vi "Tag-Get Tag.vi"(8 "error in (no error)":errorcluster, 10 "Tag Name":string, 11 "Generic in":refnum<class "Generic.lvclass">) -> (0 "error out":errorcluster, 1 "Is Persistent?":bool, 2 "Tag:Get Tag":bool, 3 "Generic out":refnum<class "Generic.lvclass">, 4 "Value":variant)   [LabVIEW 2015, in "Generic.lvclass"]
doc: "Returns a tag value associated with the tag. Returns FALSE if the tag does not exist.\n\nQControl Class wrapper around the <b>Generic : Tag:Get Tag Method</b>.\n<b> </b> <b> </b>\n©2016 Q Software Innovations, LLC (QSI)\nwritten by Quentin Alldredge\nproduced in LabVIEW 2015\n\nsupport@qsoftwareinnovations.com\nwww.qsoftwareinnovations.com\n\nAll rights reserved.\n\nRedistribution and use in source and binary forms, with or without modification, are permitted provided that the following conditions are met:\n\n * Redistributions of source code must retain the above copyright notice, this list of conditions and the following disclaimer.\n * Redistributions in binary form must reproduce the above copyright notice, this list of conditions and the following disclaimer in the documentation and/or other materials provided with the distribution.\n * Neither the name of Q Software Innovations, LLC. nor the names of its contributors may be used to endorse or promote products derived from this software without specific prior written permission.\n\nTHIS SOFTWARE IS PROVIDED BY THE COPYRIGHT HOLDERS AND CONTRIBUTORS \"AS IS\" AND ANY EXPRESS OR IMPLIED WARRANTIES, INCLUDING, BUT NOT LIMITED TO, THE IMPLIED WARRANTIES OF MERCHANTABILITY AND FITNESS FOR A PARTICULAR PURPOSE ARE DISCLAIMED. IN NO EVENT SHALL THE COPYRIGHT OWNER OR CONTRIBUTORS BE LIABLE FOR ANY DIRECT, INDIRECT, INCIDENTAL, SPECIAL, EXEMPLARY, OR CONSEQUENTIAL DAMAGES (INCLUDING, BUT NOT LIMITED TO, PROCUREMENT OF SUBSTITUTE GOODS OR SERVICES; LOSS OF USE, DATA, OR PROFITS; OR BUSINESS INTERRUPTION) HOWEVER CAUSED AND ON ANY THEORY OF LIABILITY, WHETHER IN CONTRACT, STRICT LIABILITY, OR TORT (INCLUDING NEGLIGENCE OR OTHERWISE) ARISING IN ANY WAY OUT OF THE USE OF THIS SOFTWARE, EVEN IF ADVISED OF THE POSSIBILITY OF SUCH DAMAGE."
uses:
  Generic.lvclass
  Generic.lvclass/Generic.ctl
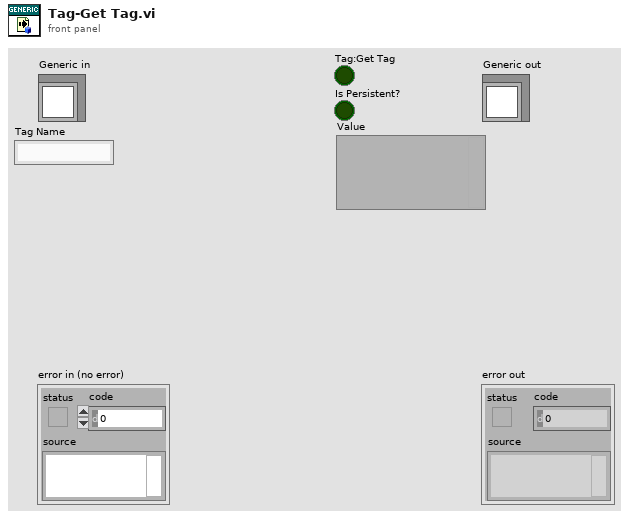
[diagram p1: front panel]
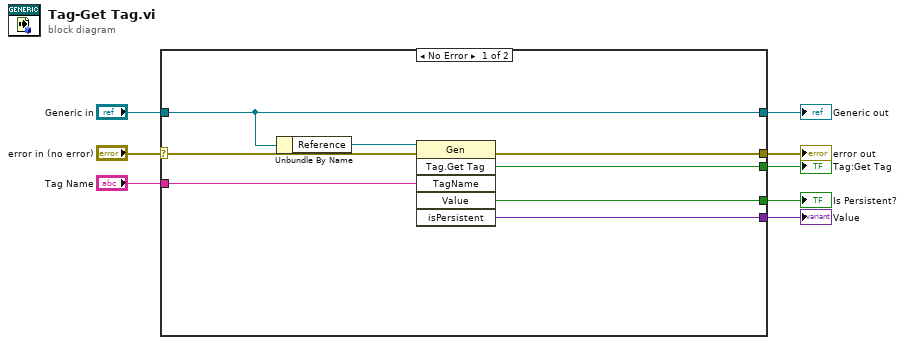
[diagram p0: block diagram]
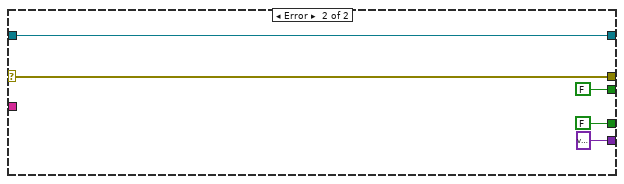
[diagram p2: hidden frame]
diagram:
  n1 = case shown="No Error" "error in (no error)" {
    selector: "error in (no error)" -> [w16 w21]
    tunnel: [w15 w21] -> w7
    tunnel: [w14 w20] -> w5
    tunnel: "Generic in" -> [w14 w20]
    tunnel: "Tag Name" -> [w12 _]
    tunnel: [w11 FALSE ("GetTag")] -> w3
    tunnel: [w10 FALSE ("Value")] -> w2
    tunnel: [w9 variant ("isPersistent")] -> w1
    frame No Error {
      n2 = Unbundle By Name(w14) -> ("Reference"=w13:refnum<vi>)
      n3 = invoke class="Gen" method="Tag.Get Tag"(reference=w13, error in=w16, "TagName"=w12) -> (error out=w15:errorcluster, "GetTag"=w11:bool, "Value"=w10:bool, "isPersistent"=w9:variant)  [unwired: 3 in, 2 out]
    }
    frame Error {
    }
  }
  "error out" <- w7
  "Generic out" <- w5
  "Tag:Get Tag" <- w3
  "Is Persistent?" <- w2
  "Value" <- w1
